vi "UDP - Discover DAQ Devices on the Network.vi"(8 "error in":errorcluster) -> (0 "Error out":errorcluster, 2 "Number of Discovered Devices":i32, 3 "List of IPs":string[](array[string]))   [LabVIEW 2021]
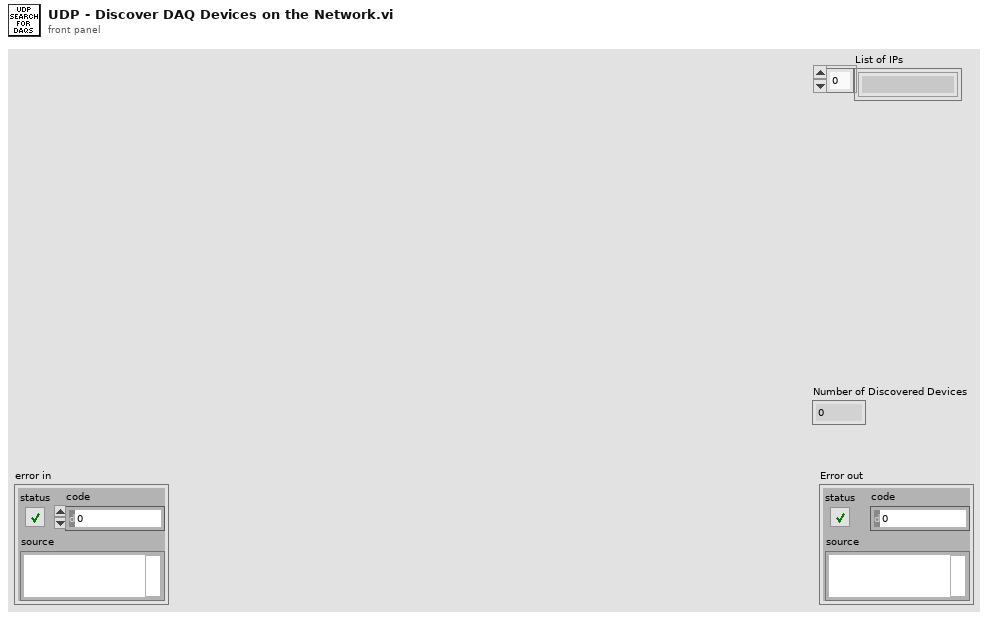
[diagram p1: front panel]
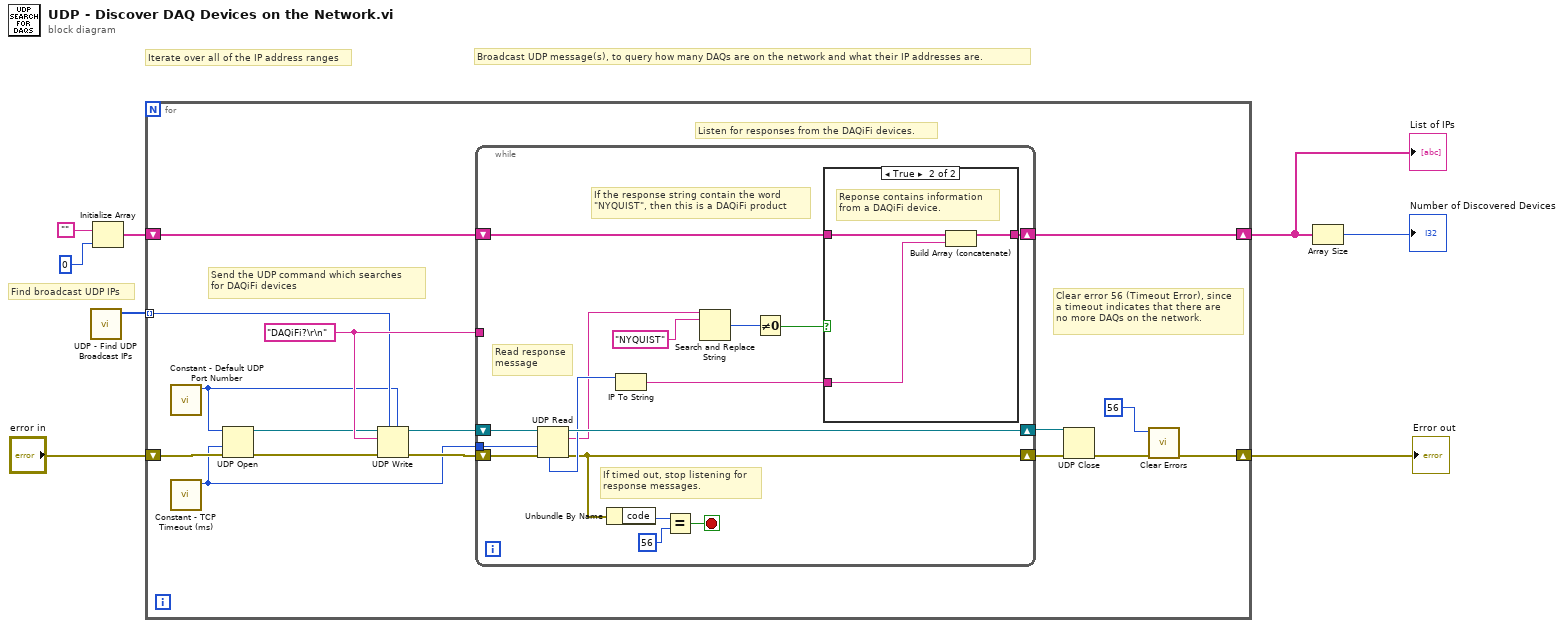
[diagram p0: block diagram]
diagram:
  # "Find broadcast UDP IPs"
  # "Iterate over all of the IP address ranges"
  # "Broadcast UDP message(s), to query how many DAQs are on the network and what their IP addresses are."
  n1 = call "UDP - Find UDP Broadcast IPs.vi"() -> ("IP Addresses"=w7:u32[])  [unwired: 11 in]
  n2 = Initialize Array("", 0 ("dimension size")) -> (w4:string[])
  n3 = for {
    shift-right: [w18] -> w2
    shift-left: "error in" -> [w16]
    tunnel: w7 -> [w11] mode=indexing
    shift-right: [w14] -> w1
    shift-left: w4 -> [w15]
    w22 = "DAQiFi?\r\n" ("data in")
    # "Listen for responses from the DAQiFi devices."
    # "Clear error 56 (Timeout Error), since\na timeout indicates that there are\nno more DAQs on the network."
    # "Send the UDP command which searches\nfor DAQiFi devices"
    n4 = call "Constant - Default UDP Port Number.vi"() -> ("port"=w9:u16)  [unwired: 11 in]
    n5 = call "Constant - TCP Timeout (ms).vi"() -> ("timeout (ms)"=w13:i32)  [unwired: 11 in]
    n6 = UDP Open(8:w16, 9:w13, 11:w9) -> (port=w12:refnum<k16>, 0:w10:errorcluster)  [unwired: 2 in, 1 out]
    n7 = UDP Write(address=w11, port or service name=w9, connection ID=w12, data in=w22, 8:w10) -> (error out=w23:errorcluster, 3:w24:refnum<k16>)  [unwired: 1 in]
    n8 = while {
      tunnel: w13 -> [w37]
      shift-right: [w38] -> w21
      shift-left: w24 -> [w40]
      shift-right: [w28] -> w20
      shift-left: w23 -> [w39]
      tunnel: w22 -> [_]
      shift-right: [w31] -> w14
      shift-left: w15 -> [w32]
      stop <- w25 stop-if-true
      # "If timed out, stop listening for\nresponse messages."
      # "If the response string contain the word\n\"NYQUIST\", then this is a DAQiFi product"
      # "Read response\nmessage"
      n9 = UDP Read(connection ID=w40, timeout ms (25000)=w37, 8:w39) -> (data out=w30:string, error out=w28:errorcluster, 3:w38:refnum<k16>, 6:w36:u32)  [unwired: 1 in, 1 out]
      n10 = Unbundle By Name(w28) -> ("code"=w27:i32)
      n11 = IP To String(2:w36) -> (0:w35:string)  [unwired: 1 in]
      n12 = Equal?(x=w27, y=56) -> (x = y?=w25:bool)
      n13 = Search and Replace String(input string=w30, search string="NYQUIST") -> (number of replacements=w33:i32)  [unwired: 6 in, 3 out]
      n14 = Not Equal To 0?(x=w33) -> (x != 0?=w29:bool)
      n15 = case shown="True" w29 {
        tunnel: w35 -> [_ w43]
        tunnel: w32 -> [w41 w44]
        tunnel: [w41 w42] -> w31
        frame False {
          # "Not a DAQifi device"
        }
        frame True {
          # "Reponse contains information\nfrom a DAQiFi device."
          n16 = Build Array (concatenate)(w44, w43) -> (w42:string[])
        }
      }
    }
    n17 = UDP Close(connection ID=w21, 8:w20) -> (error out=w19:errorcluster)  [unwired: 1 out]
    n18 = call <vilib>:"Clear Errors.vi"("error in (no error)"=w19, "specific error code to clear (0: all)"=56) -> ("error out"=w18:errorcluster)  [unwired: 4 in, 1 out]
  }
  "Error out" <- w2
  "List of IPs" <- w1
  n19 = Array Size(array=w1) -> (size(s)=→"Number of Discovered Devices":i32)
